vi "Cube Drop.vi"   [LabVIEW 2020, in "VolatusGUIElements.lvlib"]
uses:
  VolatusGUIElements.lvlib
  NumericIndicator/NumericIndicator.lvclass
  DblNumericStatusIndicator/DblStatusIndicator.lvclass
  LocalGraphBuffer/LocalGraphBuffer.lvclass
  2WayValveV/2WayValveV.lvclass
  2WayValveH/2WayValveH.lvclass
  LoggingControl/LoggingControl.lvclass
  DblPopupControl/DblPopupControl.lvclass
  DigitalButtonControl/DigitalButtonControl.lvclass
  BooleanIndicator/BooleanIndicator.lvclass
  DoubleControl/SliderControl.lvclass
  SystemConfigStatusIndicator/SystemConfigStatusIndicator.lvclass
  NumericRangeBooleanIndicator/NumericRangeBooleanIndicator.lvclass
  GroupLoggingControl/GroupLoggingControl.lvclass
  ImageButtonControl/ImageButtonControl.lvclass
  BooleanControl/BooleanControl.lvclass
  BluelinesRedlines/BluelinesRedlines.lvclass
  GaugeIndicator/GaugeIndicator.lvclass
  HistorianCharting/HistorianCharting.lvclass
  VolatusGUI/VolatusGUI.lvlib
  GuiLinkButton/GuiLinkButton.lvclass
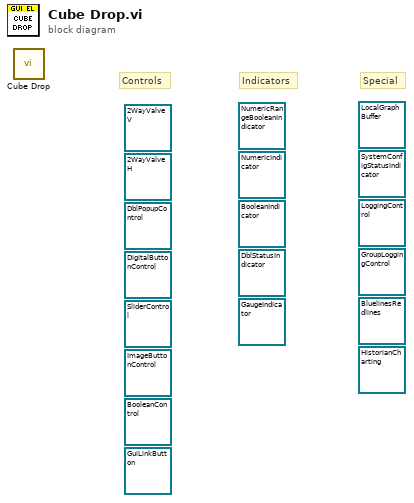
[diagram p0: block diagram]
diagram:
  (unwired) refnum<class "GuiLinkButton.lvclass"> refnum ("VolatusGUIElements.lvlib:GuiLinkButton.lvclass")
  (unwired) refnum<class "HistorianCharting.lvclass"> refnum ("VolatusGUIElements.lvlib:HistorianCharting.lvclass")
  (unwired) refnum<class "GaugeIndicator.lvclass"> refnum ("VolatusGUIElements.lvlib:GaugeIndicator.lvclass")
  (unwired) refnum<class "BluelinesRedlines.lvclass"> refnum ("VolatusGUIElements.lvlib:BluelinesRedlines.lvclass")
  (unwired) refnum<class "BooleanControl.lvclass"> refnum ("VolatusGUIElements.lvlib:BooleanControl.lvclass")
  (unwired) refnum<class "ImageButtonControl.lvclass"> refnum ("VolatusGUIElements.lvlib:ImageButtonControl.lvclass")
  (unwired) refnum<class "GroupLoggingControl.lvclass"> refnum ("VolatusGUIElements.lvlib:GroupLoggingControl.lvclass")
  (unwired) refnum<class "NumericRangeBooleanIndicator.lvclass"> refnum ("VolatusGUIElements.lvlib:NumericRangeBooleanIndicator.lvclass")
  (unwired) refnum<class "SystemConfigStatusIndicator.lvclass"> refnum ("VolatusGUIElements.lvlib:SystemConfigStatusIndicator.lvclass")
  (unwired) refnum<class "SliderControl.lvclass"> refnum ("VolatusGUIElements.lvlib:SliderControl.lvclass")
  (unwired) refnum<class "BooleanIndicator.lvclass"> refnum ("VolatusGUIElements.lvlib:BooleanIndicator.lvclass")
  (unwired) refnum<class "DigitalButtonControl.lvclass"> refnum ("VolatusGUIElements.lvlib:DigitalButtonControl.lvclass")
  (unwired) refnum<class "DblPopupControl.lvclass"> refnum ("VolatusGUIElements.lvlib:DblPopupControl.lvclass")
  (unwired) refnum<class "LoggingControl.lvclass"> refnum ("VolatusGUIElements.lvlib:LoggingControl.lvclass")
  (unwired) refnum<class "2WayValveH.lvclass"> refnum ("VolatusGUIElements.lvlib:2WayValveH.lvclass")
  (unwired) refnum<class "2WayValveV.lvclass"> refnum ("VolatusGUIElements.lvlib:2WayValveV.lvclass")
  (unwired) refnum<class "LocalGraphBuffer.lvclass"> refnum ("VolatusGUIElements.lvlib:LocalGraphBuffer.lvclass")
  (unwired) refnum<class "DblStatusIndicator.lvclass"> refnum ("VolatusGUIElements.lvlib:DblStatusIndicator.lvclass")
  (unwired) refnum<class "NumericIndicator.lvclass"> refnum ("VolatusGUIElements.lvlib:NumericIndicator.lvclass")
  # "Special"
  # "Indicators"
  # "Controls"
  n1 = call "Cube Drop.vi"() -> ()  [unwired: 12 in]
